vi "Analyze Cache Size.vi"(8 "error in (no error)":errorcluster, 11 "DataSize":i32) -> (0 "error out":errorcluster, 3 "CacheSize":i32)   [LabVIEW 2017, in "MDPtr.lvlib" / "MDPtrMgr.lvclass"]
uses:
  MDPtrMgr.lvclass
  MDPtr.lvlib
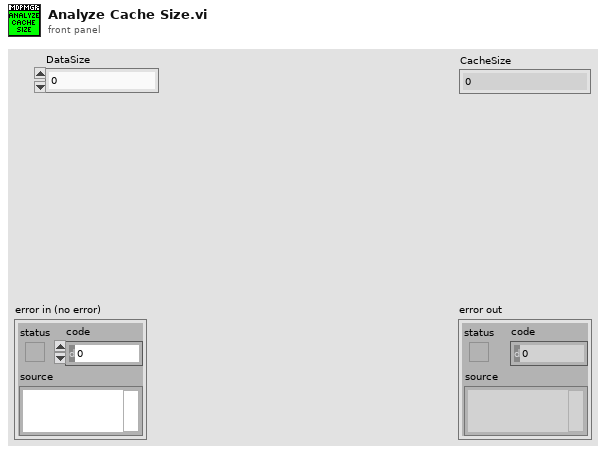
[diagram p1: front panel]
types:
  T1 = typedef "MDPtr.lvlib/MDPtr GlobalSettings.ctl" = cluster{"Malloc Method":T2, "FixedPreSize":cluster{"PreCacheSize":i32}}
  T2 = typedef "MDPtr.lvlib/MDPtr MallocMethod.ctl" = enum16{"NONE", "FIXED PRE-SIZE"}
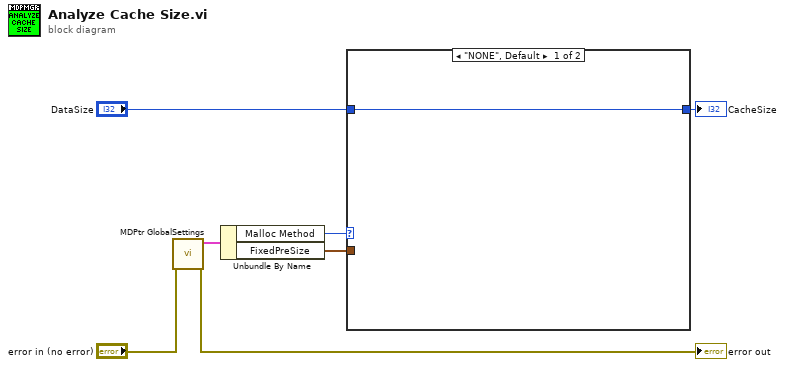
[diagram p0: block diagram]
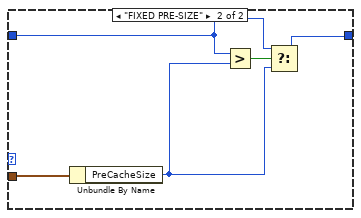
[diagram p2: hidden frame]
diagram:
  n1 = call "MDPtr GlobalSettings.vi"("error in (no error)"="error in (no error)") -> ("error out"=→"error out":errorcluster, "Setting out"=w7:T1)  [unwired: 9 in]
  n2 = Unbundle By Name(w7) -> ("Malloc Method"=w6:T2, "FixedPreSize"=w1:cluster{"PreCacheSize":i32})
  n3 = case shown="\"NONE\", Default" w6 {
    tunnel: [w8 w10] -> w5
    tunnel: "DataSize" -> [w8 w12]
    tunnel: w1 -> [_ w13]
    frame "NONE", Default {
    }
    frame "FIXED PRE-SIZE" {
      n4 = Unbundle By Name(w13) -> ("PreCacheSize"=w11:i32)
      n5 = Greater?(x=w12, y=w11) -> (0:w9:bool)
      n6 = Select(t=w12, s=w9, f=w11) -> (s? t:f=w10:i32)
    }
  }
  "CacheSize" <- w5
